vi "Convert Homography to Pose.vi"(6 "filter":T1, 9 "Scale to Inches":dbl[](array[numeric])=[-2.8, 1.0, 4.1], 10 "Inverse Camera Matrix":T3, 11 "tag info":T2={"tag ID"=0, "Center (pix)"={"X"=0.0, "Y"=0.0}, "homography matrix"=[], "score"=0.0, "Hamming Dist"=0, "corners (pix)"=[], "Tag Family"="36h11"}) -> (1 "Translation":dbl[](array[numeric]), 2 "angles SVD":cluster{"yaw":dbl, "pitch":dbl, "roll":dbl}, 3 "angles (deg)":cluster{"yaw":dbl, "pitch":dbl, "roll":dbl})   [LabVIEW 2025]
uses:
  <vilib>/Analysis/Matrix/Datatypes/RealMatrix.ctl
  filter Selector.ctl
  <vilib>/Analysis/7linalg.llb/SVD Option.ctl
  <vilib>/Analysis/baseanly.llb/Real A x B.vi
  <vilib>/Analysis/_algsub.llb/Real Vector Norm.vi
  <vilib>/Analysis/7linalg.llb/Real Transpose Matrix.vi
  <vilib>/Analysis/baseanly.llb/A x Vector.vi
  <vilib>/Analysis/Matrix/Numeric/Multiply/Multiply - R,RM.vi
  <vilib>/addons/control/pid/pid.llb/PID Control Input Filter (DBL Array).vi
  <vilib>/Analysis/7linalg.llb/Real SVD Decomposition.vi
  <vilib>/Analysis/NI_AALBase.lvlib
  <vilib>/Analysis/NI_AALPro.lvlib
  <vilib>/robotics/Kinematics/NI_Kinematics.lvlib
  <vilib>/Analysis/Matrix/NI_Matrix.lvlib
  <vilib>/addons/control/pid/NI_PID_pid.lvlib
  <vilib>/ptbypt/NI_PtbyPt.lvlib
panel:
  in  "median rank":i32=1
  out "raw translation":dbl[](array[numeric])
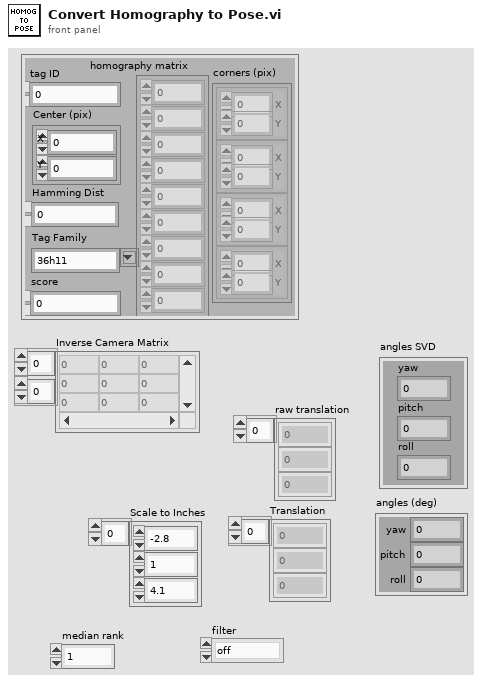
[diagram p1: front panel]
types:
  T1 = typedef "filter Selector.ctl" = enum16{"off", "2 pt avg", "low pass"}
  T2 = cluster{"tag ID":i32, "Center (pix)":cluster{"X":dbl, "Y":dbl}, "homography matrix":dbl[], "score":dbl, "Hamming Dist":i32, "corners (pix)":cluster{"X":dbl, "Y":dbl}[], "Tag Family":string}
  T3 = typedef "NI_Matrix.lvlib/RealMatrix.ctl" = dbl[][]
  T4 = typedef "NI_AALPro.lvlib/SVD Option.ctl" = u16
  T5 = cluster{"Filtered x":dbl, "Filtered x":dbl, "Filtered x":dbl}
  T6 = cluster{"output[0]":dbl, "output[1]":dbl, "output[2]":dbl}
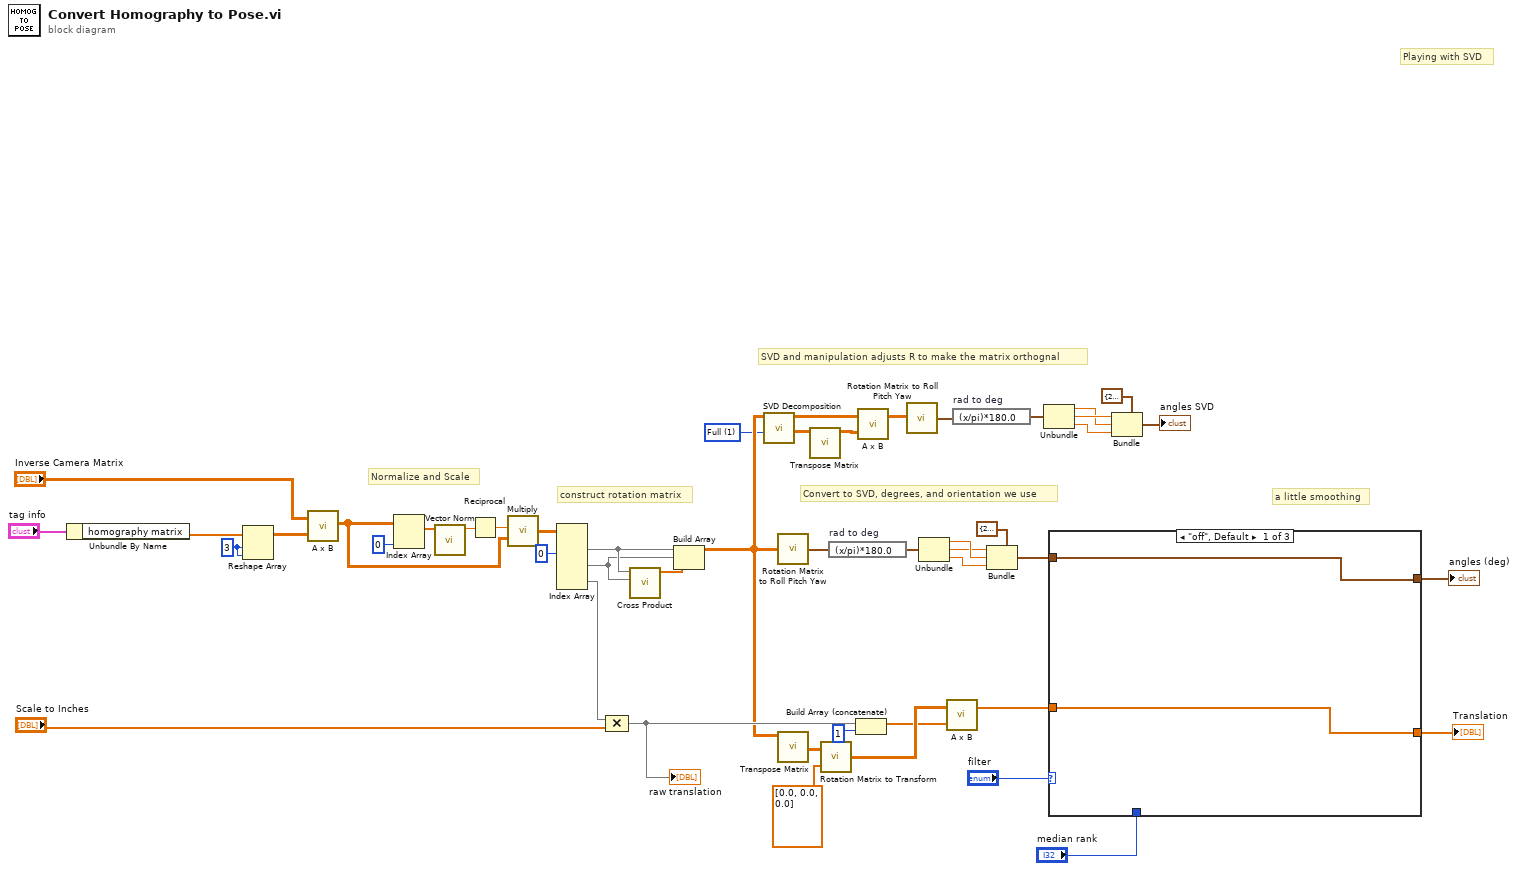
[diagram p0: block diagram]
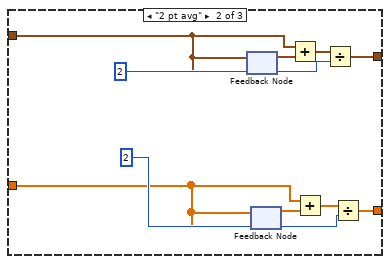
[diagram p2: hidden frame]
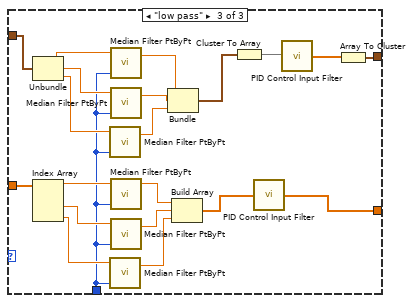
[diagram p3: hidden frame]
diagram:
  w10 = T4 1 items=["Thin", "Full"] ("SVD option")
  w48 = 3 ("dimension size")
  # "SVD and manipulation adjusts R to make the matrix orthognal"
  # "a little smoothing"
  # "Convert to SVD, degrees, and orientation we use"
  # "construct rotation matrix"
  # "Normalize and Scale"
  # "Playing with SVD"
  n1 = Unbundle By Name("tag info") -> ("homography matrix"=w16:dbl[])
  n2 = Reshape Array(w16, w48, w48) -> (w15:dbl[][])
  n3 = call-poly <vilib>:"A x B.vi"("B"=w15, "A"="Inverse Camera Matrix") -> ("A x B"=w42:T3)  [unwired: 1 out]
  n4 = Index Array(array=w42, index (col)=0 ("disabled index (col)")) -> (element=w44:dbl[])  [unwired: 1 in]
  n5 = call-poly <vilib>:"Vector Norm.vi"("Input Vector"=w44) -> ("norm"=w45:dbl)  [unwired: 9 in, 1 out]
  n6 = Reciprocal(x=w45) -> (1/x=w43:dbl)
  n7 = call-poly <vilib>:"Multiply.vi"("Real Matrix A"=w42, "Real Scalar c"=w43) -> ("c * A"=w40:T3)
  n8 = Index Array(array=w40, index (col) #1=0 ("disabled index (col)")) -> (element #1=w39:dbl[], element #2=w38:dbl[], element #3=w30:dbl[])  [unwired: 5 in]
  n9 = Compound Arithmetic op=MULTIPLY(w30, "Scale to Inches") -> (w27:dbl[])
  "raw translation" <- w27
  n10 = call <vilib>:"Cross Product.vi"("B Vector"=w38, "A Vector"=w39) -> ("Cross Product"=w37:dbl[])  [unwired: 8 in, 1 out]
  n11 = Build Array(w39, w38, w37) -> (w23:T3)
  n12 = call-poly <vilib>:"SVD Decomposition.vi"("SVD option"=w10, "A"=w23) -> ("Matrix V"=w8:T3, "Matrix U"=w12:T3)  [unwired: 5 in, 3 out]
  n13 = call <vilib>:"Rotation Matrix to Roll Pitch Yaw.vi"("rotation matrix"=w23) -> ("angles"=w29:cluster{"roll":dbl, "pitch":dbl, "yaw":dbl})
  n14 = call-poly <vilib>:"Transpose Matrix.vi"("Input Matrix"=w23) -> ("Matrix Transpose"=w22:T3)  [unwired: 9 in, 1 out]
  n15 = call-poly <vilib>:"Transpose Matrix.vi"("Input Matrix"=w8) -> ("Matrix Transpose"=w7:T3)  [unwired: 9 in, 1 out]
  n16 = call <vilib>:"Rotation Matrix to Transform.vi"("translation vector"=dbl[] [0.0, 0.0, 0.0] ("subarray"), "rotation matrix"=w22) -> ("transform"=w28:T3)
  n17 = expression code="(x/pi)*180.0" "rad to deg"(w29) -> (w32:cluster{"roll":dbl, "pitch":dbl, "yaw":dbl})
  n18 = Build Array (concatenate)(w27, 1 ("dimension size")) -> (w24:dbl[])
  n19 = call-poly <vilib>:"A x B.vi"("B"=w7, "A"=w12) -> ("A x B"=w9:T3)  [unwired: 1 out]
  n20 = call <vilib>:"Rotation Matrix to Roll Pitch Yaw.vi"("rotation matrix"=w9) -> ("angles"=w11:cluster{"roll":dbl, "pitch":dbl, "yaw":dbl})
  n21 = Unbundle(w32) -> ("roll"=w36:dbl, "pitch"=w33:dbl, "yaw"=w35:dbl)
  n22 = call-poly <vilib>:"A x B.vi"("Vector"=w24, "A"=w28) -> ("A x Vector"=w19:dbl[])  [unwired: 1 out]
  n23 = expression code="(x/pi)*180.0" "rad to deg"(w11) -> (w2:cluster{"roll":dbl, "pitch":dbl, "yaw":dbl})
  n24 = Bundle(cluster=cluster{"yaw":dbl, "pitch":dbl, "roll":dbl} {"yaw"=25.18811270112165, "pitch"=-30.885572547805758, "roll"=-2.4619221233355195} ("YPR (deg)"), "yaw"=w33, "pitch"=w36, "roll"=w35) -> (w21:cluster{"yaw":dbl, "pitch":dbl, "roll":dbl})
  n25 = Unbundle(w2) -> ("roll"=w3:dbl, "pitch"=w6:dbl, "yaw"=w4:dbl)
  n26 = case shown="\"off\", Default" "filter" {
    tunnel: w21 -> [w50 w54 w70]
    tunnel: [w50 w53 w78] -> w20
    tunnel: w19 -> [w49 w52 w69]
    tunnel: [w49 w51 w81] -> w18
    tunnel: "median rank" -> [_ _ w61]
    frame "off", Default {
    }
    frame "2 pt avg" {
      n27 = feedback #1(w54) -> (w59:cluster{"yaw":dbl, "pitch":dbl, "roll":dbl})
      n28 = feedback-in #1(w54) -> ()
      n29 = feedback #2(w52) -> (w60:dbl[])
      n30 = feedback-in #2(w52) -> ()
      n31 = Add(x=w54, y=w59) -> (x+y=w58:cluster{"yaw":dbl, "pitch":dbl, "roll":dbl})
      n32 = Add(x=w52, y=w60) -> (x+y=w57:dbl[])
      n33 = Divide(x=w58, y=2 ("disabled index (col)")) -> (x/y=w53:cluster{"yaw":dbl, "pitch":dbl, "roll":dbl})
      n34 = Divide(x=w57, y=2 ("disabled index (col)")) -> (x/y=w51:dbl[])
    }
    frame "low pass" {
      n35 = Unbundle(w70) -> ("yaw"=w77:dbl, "pitch"=w76:dbl, "roll"=w75:dbl)
      n36 = Index Array(array=w69) -> (element #1=w68:dbl, element #2=w67:dbl, element #3=w66:dbl)  [unwired: 3 in]
      n37 = call <vilib>:"Median Filter PtByPt.vi"("rank"=w61, "x"=w75) -> ("Filtered x"=w72:dbl)  [unwired: 2 in, 1 out]
      n38 = call <vilib>:"Median Filter PtByPt.vi"("rank"=w61, "x"=w66) -> ("Filtered x"=w63:dbl)  [unwired: 2 in, 1 out]
      n39 = call <vilib>:"Median Filter PtByPt.vi"("rank"=w61, "x"=w77) -> ("Filtered x"=w74:dbl)  [unwired: 2 in, 1 out]
      n40 = call <vilib>:"Median Filter PtByPt.vi"("rank"=w61, "x"=w76) -> ("Filtered x"=w73:dbl)  [unwired: 2 in, 1 out]
      n41 = call <vilib>:"Median Filter PtByPt.vi"("rank"=w61, "x"=w68) -> ("Filtered x"=w65:dbl)  [unwired: 2 in, 1 out]
      n42 = call <vilib>:"Median Filter PtByPt.vi"("rank"=w61, "x"=w67) -> ("Filtered x"=w64:dbl)  [unwired: 2 in, 1 out]
      n43 = Bundle("Filtered x"=w74, "Filtered x"=w73, "Filtered x"=w72) -> (w71:T5)  [unwired: 1 in]
      n44 = Build Array(w65, w64, w63) -> (w62:dbl[])
      n45 = Cluster To Array(cluster=w71) -> (array=w80:dbl[])
      n46 = call-poly <vilib>:"PID Control Input Filter.vi"("input"=w62) -> ("output"=w81:dbl[])  [unwired: 4 in]
      n47 = call-poly <vilib>:"PID Control Input Filter.vi"("input"=w80) -> ("output"=w79:dbl[])  [unwired: 4 in]
      n48 = Array To Cluster(array=w79) -> (cluster=w78:T6)
    }
  }
  "angles (deg)" <- w20
  "Translation" <- w18
  n49 = Bundle(cluster=cluster{"yaw":dbl, "pitch":dbl, "roll":dbl} {"yaw"=25.18811270112165, "pitch"=-30.885572547805758, "roll"=-2.4619221233355195} ("YPR (deg)"), "yaw"=w6, "pitch"=w3, "roll"=w4) -> (→"angles SVD":cluster{"yaw":dbl, "pitch":dbl, "roll":dbl})
